vi "Read Message from Tool.vi"(8 "error in (no error)":errorcluster) -> (0 "error out":errorcluster, 1 "timed out?":bool, 2 "Message Data":variant, 3 "Message":string)   [LabVIEW 2015, in "Tool Interface.lvlib"]
uses:
  Tool Interface.lvlib
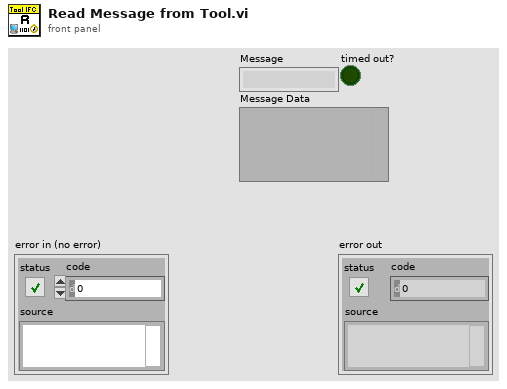
[diagram p1: front panel]
types:
  T1 = typedef "Message Cluster.ctl" = cluster{"Message":string, "Message Data":variant}
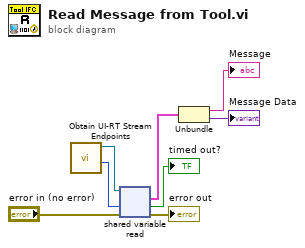
[diagram p0: block diagram]
diagram:
  n1 = call "Obtain UI-RT Stream Endpoints.vi"() -> ("Connect Timeout(ms)"=w1:i32, "RT Message Stream"=w6:refnum<k21>)  [unwired: 9 in, 1 out]
  n2 = shared-variable-read(w6, "error in (no error)", w1) -> (→"error out":errorcluster, →"timed out?":bool, w5:T1)  [unwired: 1 out]
  n3 = Unbundle(w5) -> ("Message"=→"Message":string, "Message Data"=→"Message Data":variant)
